vi "XY Graph Smoothen Plot Tail.vi"(8 "error in (no error)":errorcluster, 9 "balance parameter (-1: auto)":dbl=-1.0, 10 "Peak index (-1: unknown)":i32=-1, 11 "Plot in":cluster{"t Array":dbl[], "Y Array":dbl[]}) -> (0 "error out":errorcluster, 3 "Plot out":cluster{"t Array":dbl[], "Y Array":dbl[]})   [LabVIEW 2021, in "XY Graph Add-Ons.lvlib"]
uses:
  XY Graph Add-Ons.lvlib
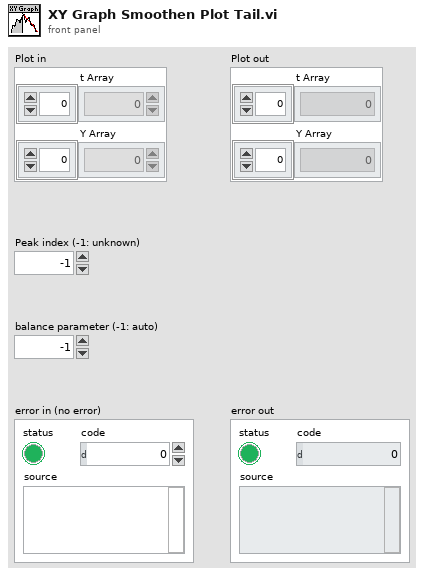
[diagram p1: front panel]
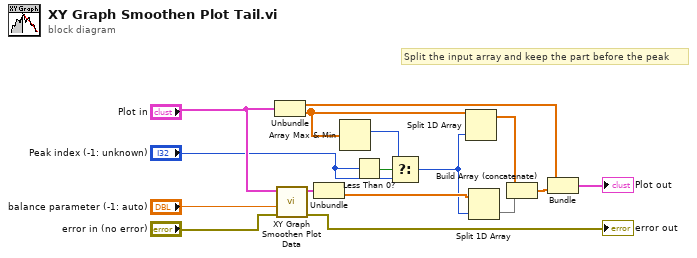
[diagram p0: block diagram]
diagram:
  # "Split the input array and keep the part before the peak"
  n1 = Unbundle("Plot in") -> ("t Array"=w13:dbl[], "Y Array"=w3:dbl[])
  n2 = call "XY Graph Smoothen Plot Data.vi"("Error In"="error in (no error)", "balance parameter (Cubic Spline, -1: auto)"="balance parameter (-1: auto)", "Plot"="Plot in") -> ("error out"=→"error out":errorcluster, "Cubic Splined Plot"=w9:cluster{"X Array":dbl[], "Y Array":dbl[]})  [unwired: 7 in]
  n3 = Unbundle(w9) -> ("Y Array"=w10:dbl[])  [unwired: 1 out]
  n4 = Array Max & Min(array=w3) -> (max index (indices)=w2:i32)  [unwired: 3 out]
  n5 = Less Than 0?(x="Peak index (-1: unknown)") -> (x < 0?=w6:bool)
  n6 = Select(t=w2, s=w6, f="Peak index (-1: unknown)") -> (s? t:f=w4:i32)
  n7 = Split 1D Array(array=w3, index=w4) -> (first subarray=w7:dbl[])  [unwired: 1 out]
  n8 = Split 1D Array(array=w10, index=w4) -> (second subarray=w8:dbl[])  [unwired: 1 out]
  n9 = Build Array (concatenate)(w7, w8) -> (w12:dbl[])
  n10 = Bundle("t Array"=w13, w12) -> (→"Plot out":cluster{"t Array":dbl[], dbl[]})  [unwired: 1 in]
